vi "PulseMinusOne.vi"(2 "error in":errorcluster, 3 "Tree Name":string="proto_tree") -> (0 "error out":errorcluster, 1 "Shot #":i32)   [LabVIEW 2014]
doc: "Finds the current MDS+ shot number, decreases the value by one, and sets the MDS+ shot number to the new value.\n\nThis, foir example, can be used to 'wipe' the shot data if the user chooses to 'Discard' shot data."
uses:
  <vilib>/MDSplus/Library/MDSplus.lvlib
  <vilib>/MDSplus/Classes/Tree_Class/Tree.lvclass
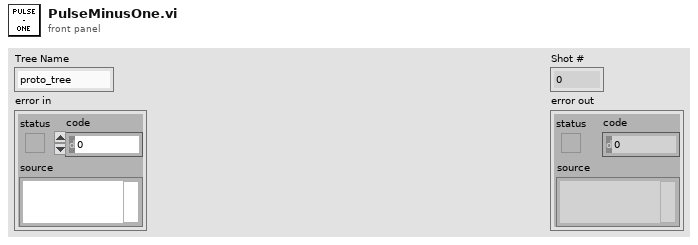
[diagram p1: front panel]
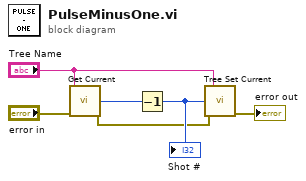
[diagram p0: block diagram]
diagram:
  n1 = call <vilib>:"Get Current.vi"("error in (no error)"="error in", "Tree name"="Tree Name") -> ("error out"=w4:errorcluster, "Current shot out"=w6:i32)  [unwired: 7 in, 1 out]
  n2 = Decrement(x=w6) -> (x-1=w5:i32)
  "Shot #" <- w5
  n3 = call <vilib>:"Tree Set Current.vi"("error in (no error)"=w4, "Shot"=w5, "Tree name"="Tree Name") -> ("error out"=→"error out":errorcluster)  [unwired: 7 in, 1 out]
